vi "MainBox To TopBox Update.vi"() -> (2 "out":T1, 3 "enqueue?":bool)   [LabVIEW 2019]
uses:
  RT Controls/Top Process Commands.ctl
  RT Controls/Top Command Events.ctl
  RT Controls/MainBox Idle.ctl
  RT Controls/Main Box Status.ctl
  RT Controls/Rotation Status.ctl
  RT Controls/Last Rotation.ctl
  RT Controls/Homing State.ctl
  RT Controls/Main Box Buttons.ctl
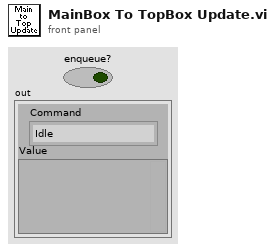
[diagram p1: front panel]
types:
  T1 = typedef "Top Process Commands.ctl" = cluster{"Command":T2, "Value":variant}
  T2 = typedef "Top Command Events.ctl" = enum16{"Idle", "FullStop", "ReadConfig", "WriteConfig", "OpenUpper", "CloseUpper", "OpenLower", "CloseLower", "SetWatchdogInt", "EnRainShutDn", "DisRainShutDn", "SetDoorMoveTO", "EnAutoShutDn", "DisAutoShutDn", "SetRevDelay", "SetRainDelay", "SyncClose", "SyncOpen"}
  T3 = typedef "MainBox Idle.ctl" = cluster{"EMButton":bool, "Shutdown":bool, "CloseMainDoor":bool, "OpenMainDoor":bool, "CloseLowerDoor":bool, "OpenLowerDoor":bool}
  T4 = typedef "Main Box Status.ctl" = cluster{"RotStatus":T5, "EMButton":bool, "TopComms":bool, "CurAZ":dbl, "At Home":bool, "LastRot":T6, "Cloud":bool, "CurAZEnc":u64, "LastAZ":dbl, "AutoShut":bool, "WDTime":bool, "HomeState":T7}
  T5 = typedef "Rotation Status.ctl" = enum16{"Stop", "Left", "Right", "Homing"}
  T6 = typedef "Last Rotation.ctl" = enum16{"--", "RR", "RL"}
  T7 = typedef "Homing State.ctl" = enum16{"Idle", "SlewFwd", "SlewRev", "SeekFwd", "SeekRev", "AtHome", "FwdWait", "RevWait"}
  T8 = typedef "Main Box Buttons.ctl" = cluster{"EMStop":bool, "CloseMainDoor":bool, "OpenMainDoor":bool, "CloseLowerDoor":bool, "OpenLowerDoor":bool, "ForwardDome":bool, "ReverseDome":bool}
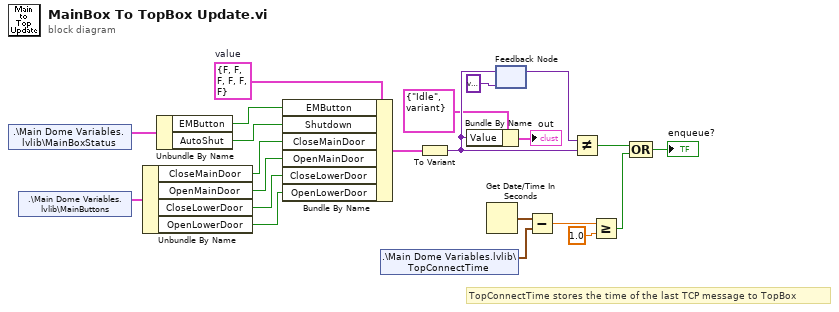
[diagram p0: block diagram]
diagram:
  w12 = T3 {"EMButton"=FALSE, "Shutdown"=FALSE, "CloseMainDoor"=FALSE, "OpenMainDoor"=FALSE, "CloseLowerDoor"=FALSE, "OpenLowerDoor"=FALSE}  # value
  # "TopConnectTime stores the time of the last TCP message to TopBox"
  n1 = shared-variable ".\\Main Dome Variables.lvlib\\MainBoxStatus"() -> (w5:T4)  [unwired: 1 in, 1 out]
  n2 = shared-variable ".\\Main Dome Variables.lvlib\\MainButtons"() -> (w4:T8)  [unwired: 1 in, 1 out]
  n3 = Unbundle By Name(w4) -> ("CloseMainDoor"=w10:bool, "OpenMainDoor"=w9:bool, "CloseLowerDoor"=w8:bool, "OpenLowerDoor"=w7:bool)
  n4 = Unbundle By Name(w5) -> ("EMButton"=w11:bool, "AutoShut"=w1:bool)
  n5 = Bundle By Name(cluster=w12, "EMButton"=w11, "Shutdown"=w1, "CloseMainDoor"=w10, "OpenMainDoor"=w9, "CloseLowerDoor"=w8, "OpenLowerDoor"=w7) -> (w6:T3)
  n6 = shared-variable ".\\Main Dome Variables.lvlib\\TopConnectTime"() -> (w17:timestamp)  [unwired: 1 in, 1 out]
  n7 = To Variant(anything=w6) -> (Variant=w22:variant)
  n8 = Bundle By Name(cluster=T1 {"Command"=enum."Idle", "Value"=variant} ("element"), "Value"=w22) -> (→"out":T1)
  n9 = Get Date/Time In Seconds() -> (seconds since 1Jan1904=w16:timestamp)
  n10 = feedback #1(variant ("Variant")) -> (w21:variant)
  n11 = feedback-in #1(w22) -> ()
  n12 = Subtract(x=w16, y=w17) -> (x-y=w15:dbl)
  n13 = Not Equal?(x=w21, y=w22) -> (x != y?=w19:bool)
  n14 = Greater Or Equal?(x=w15, y=1.0) -> (x >= y?=w13:bool)
  n15 = Compound Arithmetic op=OR(w19, w13) -> (→"enqueue?":bool)
